vi "Agilent 33XXX Series Generate Standard Waveform.vi"() -> ()   [LabVIEW 2010]
doc: "Shows how to generate a standard waveform."
uses:
  <instrlib>/Agilent 33XXX Series/Agilent 33XXX Series.lvlib
panel:
  in  "Frequency (1000 Hz)":dbl=1000.0
  in  "Waveform Function (1: Sine)":u16(ring)=1 items=["DC", "Sine", "Square", "Triangle", "Ramp", "Pulse", "Noise", "Sinc", "Negative Ramp", "Exponential Rise", "Exponential Fall", "Cardiac"]
  in  "Serial Configuration":T1={"Baud Rate"=9600, "Parity"=0, "Data Bits"=8, "Flow Control"=4} {"Flow Control" items=["None", "XON/XOFF", "RTS/CTS", "XON/XOFF & RTS/CTS", "DTR/DSR", "XON/XOFF & DTR/DSR"]; "Data Bits" items=["7"=7, "8"=8]; "Parity" items=["None", "Odd", "Even", "Mark", "Space"]; "Baud Rate" items=["300"=300, "600"=600, "1200"=1200, "2400"=2400, "4800"=4800, "9600"=9600, "19200"=19200]}
  in  "DC Offset (0.00 V)":dbl
  in  "Amplitude (1 Vpp)":dbl=1.0
  in  "VISA resource name":refnum<visa-resource-name>
  # "(c) 2008 National Instruments.  ALL RIGHTS RESERVED."
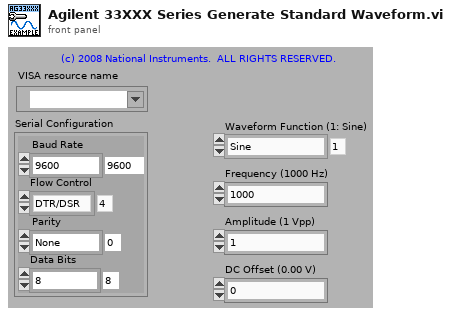
[diagram p1: front panel]
types:
  T1 = cluster{"Baud Rate":u32, "Parity":u16, "Data Bits":u16, "Flow Control":u16}
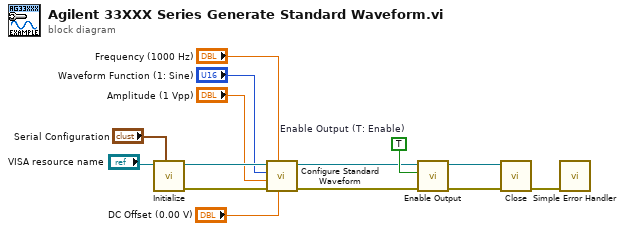
[diagram p0: block diagram]
diagram:
  w6 = TRUE  # Enable Output (T: Enable)
  n1 = call <instrlib>:"Initialize.vi"("Serial Configuration"="Serial Configuration", "VISA resource name"="VISA resource name") -> ("error out"=w12:errorcluster, "VISA resource name out"=w13:refnum<visa-resource-name>)  [unwired: 8 in]
  n2 = call <instrlib>:"Configure Standard Waveform.vi"("DC Offset (0.00 V)"="DC Offset (0.00 V)", "Frequency (1000 Hz)"="Frequency (1000 Hz)", "error in (no error)"=w12, "Amplitude (1)"="Amplitude (1 Vpp)", "Waveform Function (1: Sine)"="Waveform Function (1: Sine)", "VISA resource name"=w13) -> ("error out"=w4:errorcluster, "VISA resource name out"=w5:refnum<visa-resource-name>)  [unwired: 4 in]
  n3 = call <instrlib>:"Enable Output.vi"("error in (no error)"=w4, "Enable Output  (T: Enable)"=w6, "VISA resource name"=w5) -> ("error out"=w2:errorcluster, "VISA resource name out"=w3:refnum<visa-resource-name>)  [unwired: 7 in]
  n4 = call <instrlib>:"Close.vi"("error in (no error)"=w2, "VISA resource name"=w3) -> ("error out"=w11:errorcluster)  [unwired: 9 in]
  n5 = call <vilib>:"Simple Error Handler.vi"("error in (no error)"=w11) -> ()  [unwired: 4 in, 5 out]
